vi "WhichIsWhich.vi"(8 "Button Values Array":bool[](array[boolean])) -> (2 "Button Values Cluster":T1)   [LabVIEW 2016]
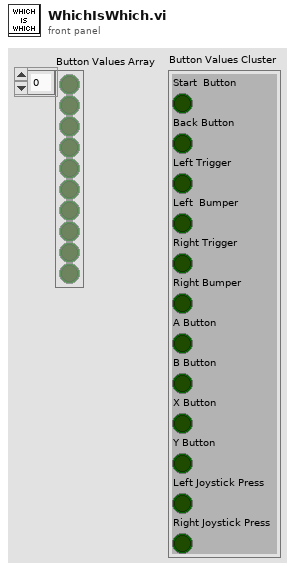
[diagram p1: front panel]
types:
  T1 = cluster{"Start  Button":bool, "Back Button":bool, "Left Trigger":bool, "Left  Bumper":bool, "Right Trigger":bool, "Right Bumper":bool, "A Button":bool, "B Button":bool, "X Button":bool, "Y Button":bool, "Left Joystick Press":bool, "Right Joystick Press":bool}
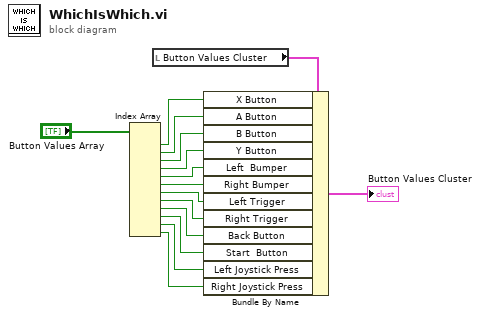
[diagram p0: block diagram]
diagram:
  n1 = Index Array(array="Button Values Array") -> (element #1=w14:bool, element #2=w13:bool, element #3=w12:bool, element #4=w11:bool, element #5=w10:bool, element #6=w9:bool, element #7=w8:bool, element #8=w7:bool, element #9=w6:bool, element #10=w5:bool, element #11=w4:bool, element #12=w3:bool)  [unwired: 12 in]
  n2 = local read "Button Values Cluster"() -> (w2:T1)
  n3 = Bundle By Name(cluster=w2, "X Button"=w14, "A Button"=w13, "B Button"=w12, "Y Button"=w11, "Left  Bumper"=w10, "Right Bumper"=w9, "Left Trigger"=w8, "Right Trigger"=w7, "Back Button"=w6, "Start  Button"=w5, "Left Joystick Press"=w4, "Right Joystick Press"=w3) -> (→"Button Values Cluster":T1)
